vi "Calibrate Ticks 2 Buttons Speed (uSMC).vi"(6 "Backlash Speed (ticks)":u16, 7 "Reset Speed (ticks)":u16=63573, 8 "Buttons Speed 4 (ticks)":u16=63573, 9 "Buttons Speed 3 (ticks)":u16=61610, 10 "Buttons Speed 2 (ticks)":u16=55720, 11 "Buttons Speed 1 (ticks)":u16=26270) -> (0 "Buttons Speed 4 (Full Steps/Sec)":u16, 1 "Buttons Speed 3 (Full Steps/Sec)":u16, 2 "Buttons Speed 2 (Full Steps/Sec)":u16, 3 "Buttons Speed 1 (Full Steps/Sec)":u16, 4 "Backlash Speed (Full Steps/Sec)":u16, 5 "Reset Speed (Full Steps/Sec)":u16)   [LabVIEW 2010, in "SignalWriterMH110203USBStepperMotor.lvclass"]
uses:
  SignalWriterMH110203USBStepperMotor.lvclass
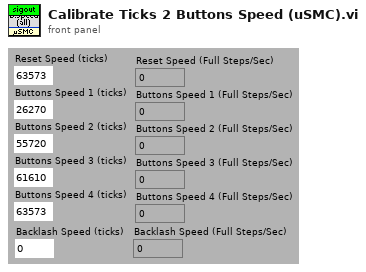
[diagram p1: front panel]
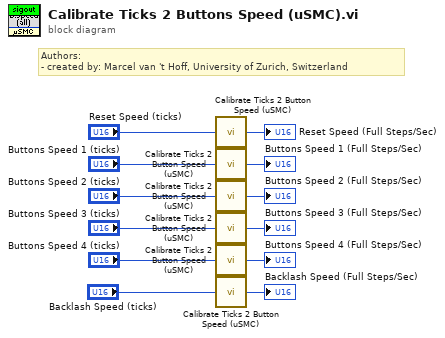
[diagram p0: block diagram]
diagram:
  # "Authors: \n- created by: Marcel van 't Hoff, University of Zurich, Switzerland"
  n1 = call "Calibrate Ticks 2 Button Speed (uSMC).vi"("Ticks"="Reset Speed (ticks)") -> ("Speed (Full Steps/Sec)"=→"Reset Speed (Full Steps/Sec)":u16)
  n2 = call "Calibrate Ticks 2 Button Speed (uSMC).vi"("Ticks"="Buttons Speed 1 (ticks)") -> ("Speed (Full Steps/Sec)"=→"Buttons Speed 1 (Full Steps/Sec)":u16)
  n3 = call "Calibrate Ticks 2 Button Speed (uSMC).vi"("Ticks"="Buttons Speed 2 (ticks)") -> ("Speed (Full Steps/Sec)"=→"Buttons Speed 2 (Full Steps/Sec)":u16)
  n4 = call "Calibrate Ticks 2 Button Speed (uSMC).vi"("Ticks"="Buttons Speed 3 (ticks)") -> ("Speed (Full Steps/Sec)"=→"Buttons Speed 3 (Full Steps/Sec)":u16)
  n5 = call "Calibrate Ticks 2 Button Speed (uSMC).vi"("Ticks"="Buttons Speed 4 (ticks)") -> ("Speed (Full Steps/Sec)"=→"Buttons Speed 4 (Full Steps/Sec)":u16)
  n6 = call "Calibrate Ticks 2 Button Speed (uSMC).vi"("Ticks"="Backlash Speed (ticks)") -> ("Speed (Full Steps/Sec)"=→"Backlash Speed (Full Steps/Sec)":u16)
